vi "Varint Decoder sint32.vi"(7 "Optional":bool, 8 "error in (no error)":errorcluster, 9 "Array":u8[](array[numeric]) format="%02x", 10 "Key":i32=-1) -> (0 "error out":errorcluster, 1 "array w/ subset deleted":u8[](array[numeric]), 2 "Read Key":i32, 3 "Varint":i32)   [LabVIEW 2020]
uses:
  Varint Decoder uint32.vi
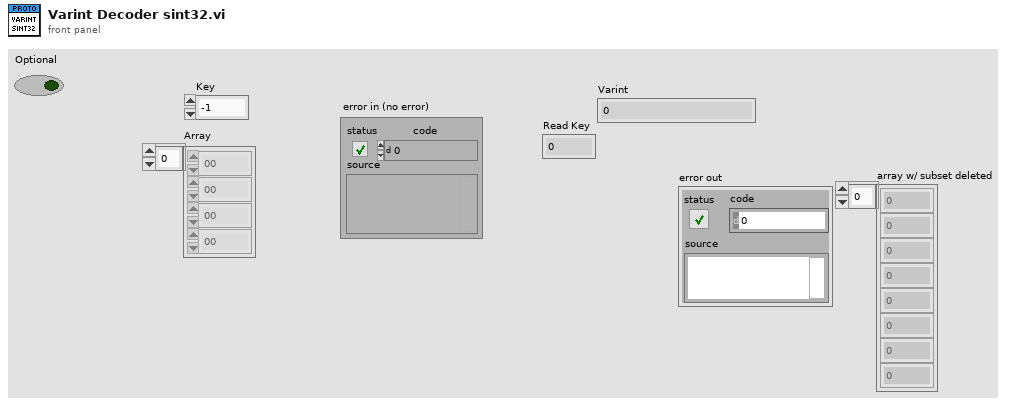
[diagram p1: front panel]
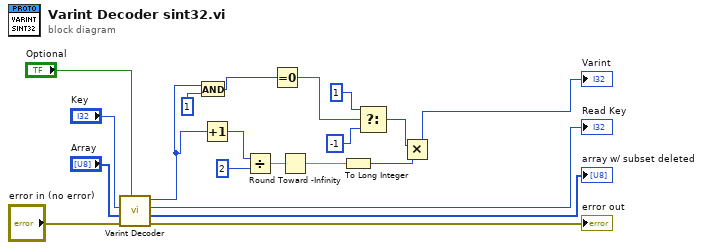
[diagram p0: block diagram]
diagram:
  n1 = call-poly "Varint Decoder.vi"("Optional"="Optional", "error in (no error)"="error in (no error)", "Array"="Array", "Key"="Key") -> ("error out"=→"error out":errorcluster, "array w/ subset deleted"=→"array w/ subset deleted":u8[], "Read Key"=→"Read Key":i32, "Varint"=w1:u32)  [unwired: 4 in]
  n2 = And(x=w1, y=u32 1) -> (x .and. y?=w10:u32)
  n3 = Increment(x=w1) -> (x+1=w13:u32)
  n4 = Divide(x=w13, y=u32 2) -> (x/y=w2:dbl)
  n5 = Equal To 0?(x=w10) -> (x = 0?=w9:bool)
  n6 = Round Toward -Infinity(1:w2) -> (0:w4:dbl)
  n7 = To Long Integer(number=w4) -> (32bit integer=w3:i32)
  n8 = Select(t=1, s=w9, f=-1) -> (s? t:f=w6:i32)
  n9 = Multiply(x=w6, y=w3) -> (x*y=→"Varint":i32)
